vi "Tests.vi"() -> ()   [LabVIEW 2022 SP3]
panel:
  out "resulting string":string
  out "output string":string
  out "Application Directory":path
  out "appended path":path
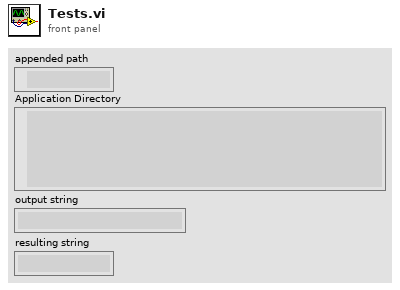
[diagram p1: front panel]
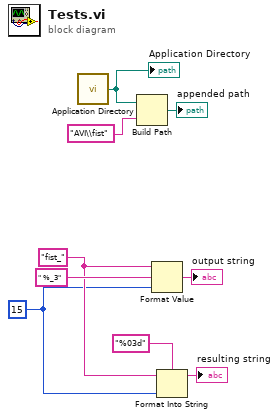
[diagram p0: block diagram]
diagram:
  w4 = "fist_" ("string (\"\")")
  w2 = u16 15 ("value (0)")
  n1 = call <vilib>:"Application Directory.vi"() -> ("Application Directory"=w9:path)
  "Application Directory" <- w9
  n2 = Build Path(base path=w9, name or relative path="AVI\\fist") -> (appended path=→"appended path":path)
  n3 = Format Value(string ("")=w4, format string=" %_3", value (0)=w2) -> (output string=→"output string":string)
  n4 = Format Into String(format string="%03d", initial string=w4, w2) -> (resulting string=→"resulting string":string)  [unwired: 1 in, 1 out]
